vi "Initialize.vi"(8 "error in (no error)":errorcluster, 9 "VISA Com Port":refnum<visa-resource-name>, 10 "Serial Device Brand":T1, 11 "Serial device in":refnum<class "Serial device.lvclass">) -> (0 "error out":errorcluster, 3 "Serial device out":refnum<class "Serial device.lvclass">)   [LabVIEW 2020, in "Serial device.lvclass"]
doc: "Metodo del papá dynamic dispatch para inicializar el dispositivo serial."
uses:
  Serial device.lvclass
  Controles/Brand combobox.ctl
  <vilib>/Instr/_visa.llb/VISA Configure Serial Port (Instr).vi
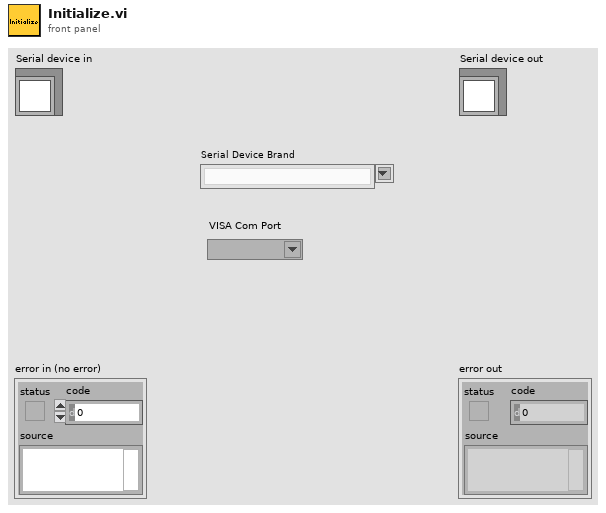
[diagram p1: front panel]
types:
  T1 = typedef "Serial device.lvclass/Brand combobox.ctl" = string
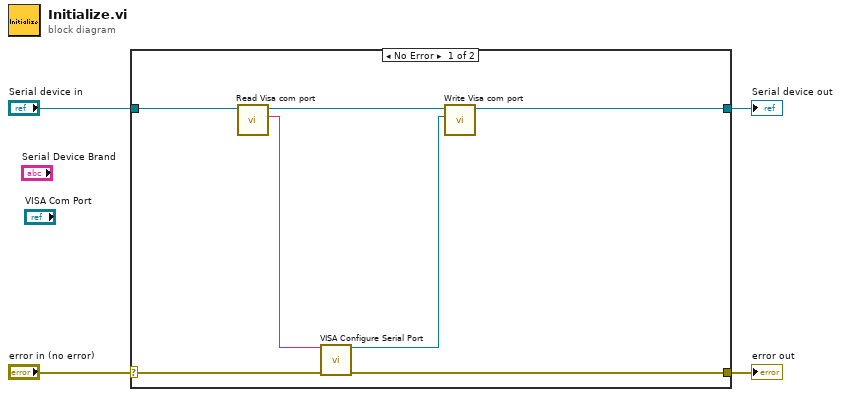
[diagram p0: block diagram]
diagram:
  n1 = case shown="No Error" "error in (no error)" {
    selector: "error in (no error)" -> [w9 w13]
    tunnel: [w8 w13] -> w3
    tunnel: [w6 w12] -> w1
    tunnel: "Serial device in" -> [w11 w12]
    frame No Error {
      n2 = call-dynamic "Read Visa com port.vi"("Serial device in"=w11) -> ("Visa com port"=w10:string, "Serial device out"=w7:refnum<class "Serial device.lvclass">)  [unwired: 8 in, 1 out]
      n3 = call-poly "VISA Configure Serial Port"("VISA resource name"=w10, "error in (no error)"=w9) -> ("VISA resource name out"=w5:refnum<visa-resource-name>, "error out"=w8:errorcluster)  [unwired: 12 in]
      n4 = call-dynamic "Write Visa com port.vi"("Visa com port"=w5, "Serial device in"=w7) -> ("Serial device out"=w6:refnum<class "Serial device.lvclass">)  [unwired: 8 in, 1 out]
    }
    frame Error {
    }
  }
  "error out" <- w3
  "Serial device out" <- w1
